vi "Add Local Chassis.vi"(8 "error in":errorcluster, 10 "settings":T2={"name"="Local Chassis", "number of slots"=8}, 11 "scan engine custom device ref in":T1 format="%.0x") -> (0 "error out":errorcluster, 1 "slot refs":T1[](array[typedef]) format="%.0x", 2 "local chassis ref":T1=18446744073709551615 format="%.0x", 3 "scan engine custom device ref out":T1 format="%.0x", 4 "user variables ref":T1=18446744073709551615 format="%.0x")   [LabVIEW 2019, in "Scan Engine Scripting.lvlib"]
doc: "Adds a local chassis to the selected Scan Engine and EtherCAT custom device."
uses:
  Scan Engine Scripting.lvlib
  Shared/Globals/Scan Engine GUIDs.vi
  Shared/SEECD Shared.lvlib
  <vilib>/NI VeriStand/Custom Device API/Custom Device API.lvlib
  Shared/Globals/Property Strings.vi
  Shared/Type Defs/Host - FPGAScanInterfaceMode.ctl
  System Explorer/SEECD System Explorer.lvlib
  Utility/Ref Constants.vi
  <vilib>/NI VeriStand/Custom Device API/Custom Device Item Ref.ctl
  Shared/Globals/Error Strings.vi
  <vilib>/NI VeriStand/Custom Device Tools/Custom Device Utility Library/Custom Device Utility Library.lvlib
  <vilib>/NI VeriStand/Custom Device Tools/Custom Device Utility Library/NI VeriStand - Search for Item by GUID.vi
  Shared/Type Defs/Local Chassis Settings.ctl
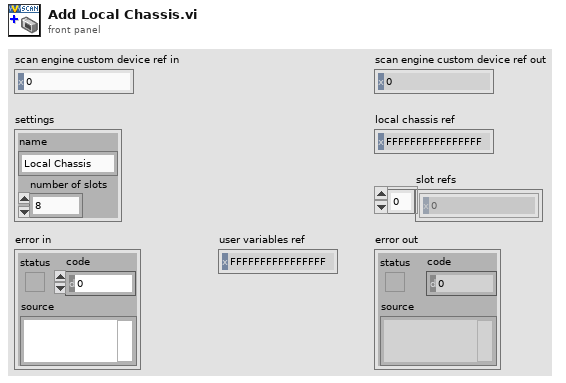
[diagram p1: front panel]
types:
  T1 = typedef "Custom Device API.lvlib/Custom Device Item Ref.ctl" = u64
  T2 = typedef "SEECD Shared.lvlib/Local Chassis Settings.ctl" = cluster{"name":string, "number of slots":i32}
  T3 = typedef "SEECD Shared.lvlib/Host - FPGAScanInterfaceMode.ctl" = enum16{"Use Current", "FPGA", "Scan Mode"}
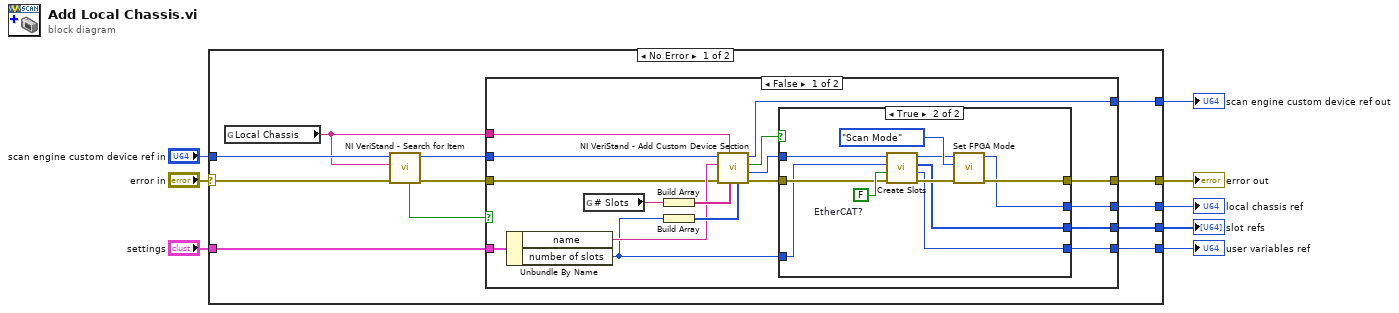
[diagram p0: block diagram]
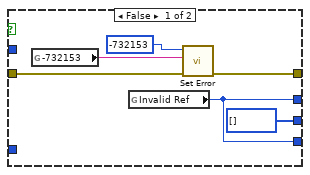
[diagram p2: hidden frame]
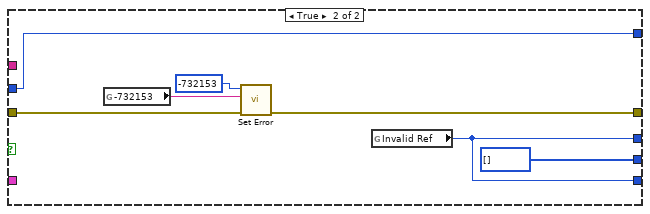
[diagram p3: hidden frame]
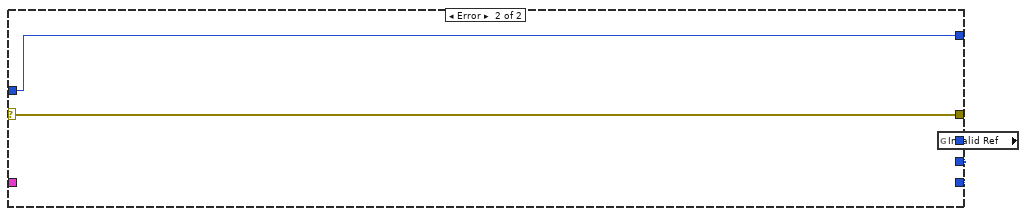
[diagram p4: hidden frame]
diagram:
  n1 = case shown="No Error" "error in" {
    selector: "error in" -> [w11 w65]
    tunnel: [w19 w65] -> w8
    tunnel: "settings" -> [w20 _]
    tunnel: "scan engine custom device ref in" -> [w14 w64]
    tunnel: [w18 w64] -> w4
    tunnel: [w15 w63] -> w3
    tunnel: [w17 T1[] [] ("slot refs")] -> w2
    tunnel: [w16 w63] -> w1
    frame No Error {
      n2 = global read "Scan Engine GUIDs.vi" "Local Chassis"() -> (w12:string)
      n3 = call-poly <vilib>:"NI VeriStand - Search for Item.vi"("error in"=w11, "Item GUID"=w12, "Section Ref in"=w14) -> ("error out"=w9:errorcluster, "Section Ref out"=w13:T1, "Found"=w10:bool)  [unwired: 5 in, 1 out]
      n4 = case shown="False" w10 {
        tunnel: w20 -> [w32 _]
        tunnel: [w29 w58] -> w19
        tunnel: [w28 w57] -> w18
        tunnel: [w26 T1[] [] ("slot refs")] -> w17
        tunnel: [w25 w56] -> w16
        tunnel: [w24 w56] -> w15
        tunnel: w13 -> [w23 w57]
        tunnel: w12 -> [w22 _]
        tunnel: w9 -> [w21 w59]
        frame False {
          n5 = Unbundle By Name(w32) -> ("name"=w31:string, "number of slots"=w30:i32)
          n6 = global read "Property Strings.vi" "# Slots"() -> (w35:string)
          n7 = Build Array(w35) -> (w36:string[])
          n8 = Build Array(w30) -> (w34:i32[])
          n9 = call <vilib>:"NI VeriStand - Add Custom Device Section.vi"("Property Values"=w34, "Property names"=w36, "GUID (Default Section)"=w22, "error in (no error)"=w21, "Section Name"=w31, "Parent Ref in"=w23) -> ("error out"=w37:errorcluster, "Section Ptr"=w27:T1, "Newly Created?"=w33:bool, "Parent Ref out"=w28:T1)  [unwired: 2 in]
          n10 = case shown="True" w33 {
            tunnel: w27 -> [_ w53]
            tunnel: w37 -> [w40 w52]
            tunnel: [w39 w50] -> w29
            tunnel: w30 -> [_ w47]
            tunnel: [T1[] [] ("slot refs") w46] -> w26
            tunnel: [w43 w45] -> w25
            tunnel: [w43 w44] -> w24
            frame False {
              n11 = global read "Error Strings.vi" "-732153"() -> (w41:string)
              n12 = global read "Ref Constants.vi" "Invalid Ref"() -> (w43:T1)
              n13 = call "Set Error.vi"("error in (no error)"=w40, "Message"=w41, "Code"=-732153 ("error code (0)")) -> ("error out"=w39:errorcluster)  [unwired: 8 in]
            }
            frame True {
              w54 = FALSE  # EtherCAT?
              n14 = call "Create Slots.vi"("error in"=w52, "EtherCAT?"=w54, "Num Slots"=w47, "Item Ref In"=w53) -> ("error out"=w51:errorcluster, "user variables ref"=w45:T1, "slot refs"=w46:T1[], "Item Ref out"=w48:T1)  [unwired: 3 in]
              n15 = call "Set FPGA Mode.vi"("error in (no error)"=w51, "FPGAScanInterfaceMode"=Host_-_FPGAScanInterfaceMode."Scan Mode", "Item Ref in"=w48) -> ("error out"=w50:errorcluster, "Item Ref out"=w44:T1)  [unwired: 7 in]
            }
          }
        }
        frame True {
          n16 = global read "Error Strings.vi" "-732153"() -> (w61:string)
          n17 = call "Set Error.vi"("error in (no error)"=w59, "Message"=w61, "Code"=-732153 ("error code (0)")) -> ("error out"=w58:errorcluster)  [unwired: 8 in]
          n18 = global read "Ref Constants.vi" "Invalid Ref"() -> (w56:T1)
        }
      }
    }
    frame Error {
      n19 = global read "Ref Constants.vi" "Invalid Ref"() -> (w63:T1)
    }
  }
  "error out" <- w8
  "scan engine custom device ref out" <- w4
  "local chassis ref" <- w3
  "slot refs" <- w2
  "user variables ref" <- w1
